vi "repmat (dbl 1d to 2d).vi"(7 "orientation":enum16{"row", "column"}(ring), 9 "c":i32=1, 10 "r":i32=1, 11 "array in":dbl[](array[numeric])) -> (3 "array out":dbl[][](array[numeric]))   [LabVIEW 2012, in "common.lvlib"]
uses:
  common.lvlib
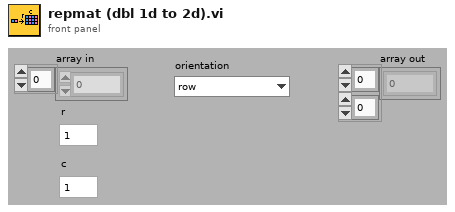
[diagram p1: front panel]
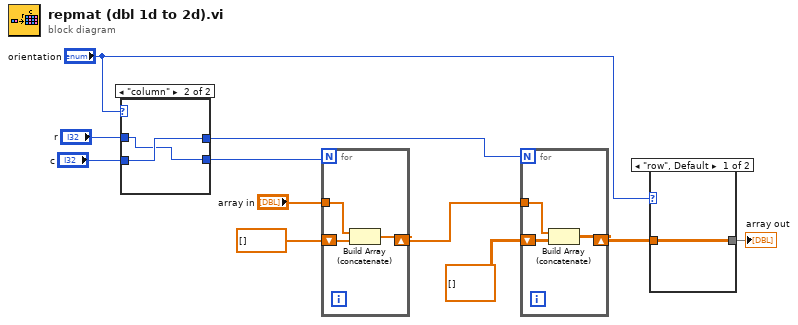
[diagram p0: block diagram]
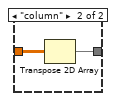
[diagram p2: hidden frame]
diagram:
  n1 = case shown="\"column\"" "orientation" {
    tunnel: "c" -> [w12 w15]
    tunnel: "r" -> [w13 w14]
    tunnel: [w13 w15] -> w2
    tunnel: [w12 w14] -> w3
    frame "row", Default {
    }
    frame "column" {
    }
  }
  n2 = for {
    N: w3 -> [_]
    tunnel: "array in" -> [w17]
    shift-right: [w16] -> w9
    shift-left: dbl[] [] ("vector") -> [w18]
    n3 = Build Array (concatenate)(w17, w18) -> (w16:dbl[])
  }
  n4 = for {
    N: w2 -> [_]
    tunnel: w9 -> [w20]
    shift-right: [w19] -> w5
    shift-left: dbl[][] [] ("vector") -> [w21]
    n5 = Build Array (concatenate)(w20, w21) -> (w19:dbl[][])
  }
  n6 = case shown="\"row\", Default" "orientation" {
    tunnel: w5 -> [w22 w24]
    tunnel: [w22 w23] -> w4
    frame "row", Default {
    }
    frame "column" {
      n7 = Transpose 2D Array(2D array=w24) -> (transposed array=w23:dbl[][])
    }
  }
  "array out" <- w4
